vi "myRIO_BRig_RT_comm_webdav_uploadFile__data.vi"(9 "input_fileName_prefix":string, 10 "input_fileName":string="dataTrial", 11 "input_hSession":T1) -> (3 "output_hSession":T1)   [LabVIEW 2014]
uses:
  <vilib>/WebDAVClient/Advanced/SessionHandle.ctl
  <vilib>/WebDAVClient/Advanced/Put File.vi
  <vilib>/WebDAVClient/NI_WebDAV.lvlib
panel:
  out "error out":errorcluster
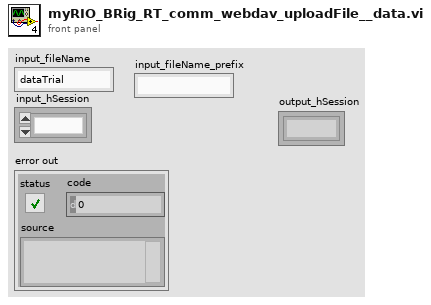
[diagram p1: front panel]
types:
  T1 = typedef "NI_WebDAV.lvlib/SessionHandle.ctl" = refnum<k1>
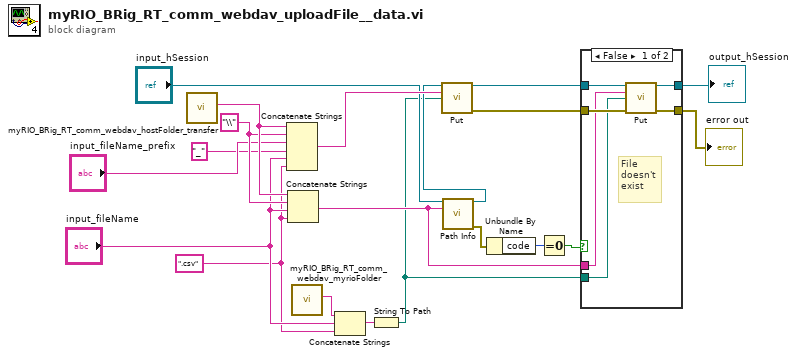
[diagram p0: block diagram]
diagram:
  w16 = "\\" ("string")
  w12 = ".csv" ("string")
  n1 = call "myRIO_BRig_RT_comm_webdav_hostFolder_transfer.vi"() -> ("output_HostFolder"=w17:string)  [unwired: 11 in]
  n2 = Concatenate Strings(w17, w16, "input_fileName_prefix", "_" ("string"), "input_fileName", w12) -> (w18:string)
  n3 = Concatenate Strings(w17, w16, "input_fileName", w12) -> (w2:string)
  n4 = call "myRIO_BRig_RT_comm_webdav_myrioFolder.vi"() -> ("output_myrioFolder"=w19:string)  [unwired: 11 in]
  n5 = Concatenate Strings(w19, "input_fileName", w12) -> (w20:string)
  n6 = String To Path(string=w20) -> (path=w1:path)
  n7 = call <vilib>:"Path Info.vi"("session handle"="input_hSession", "relative uri"=w2) -> ("session handle out"=w8:T1, "error out"=w7:errorcluster)  [unwired: 10 in, 2 out]
  n8 = call-poly <vilib>:"Put.vi"("session handle"=w8, "relative uri"=w18, "local file path"=w1) -> ("session handle out"=w6:T1, "error out"=w5:errorcluster)  [unwired: 10 in, 1 out]
  n9 = Unbundle By Name(w7) -> ("code"=w10:i32)
  n10 = Equal To 0?(x=w10) -> (x = 0?=w9:bool)
  n11 = case shown="False" w9 {
    tunnel: w6 -> [w26 w28]
    tunnel: w5 -> [w24 w27]
    tunnel: [w25 w28] -> w4
    tunnel: [w23 w27] -> w3
    tunnel: w2 -> [w22 _]
    tunnel: w1 -> [w21 _]
    frame False {
      # "File\ndoesn't\nexist"
      n12 = call-poly <vilib>:"Put.vi"("session handle"=w26, "relative uri"=w22, "local file path"=w21, "error in (no error)"=w24) -> ("session handle out"=w25:T1, "error out"=w23:errorcluster)  [unwired: 9 in, 1 out]
    }
    frame True {
      # "File\nexists"
    }
  }
  "error out" <- w3
  "output_hSession" <- w4
